vi "Funct img modulation core.vi"(8 "Pockels stay ON for at least this number of us after dwell time":dbl, 9 "Pockels turn ON at least this number of us before fill time completion":dbl, 11 "ROI setup":T1[](array[typedef]) {"Apparent Frame Size" format="%#_6f"; "Original FOV (um)" format="%#_6f"; "Pixels per miniscan" format="%#_6f"; "Dwell Time per pixel" format="%#_6f"; "Resolution" format="%#_6f"; "ROI group ID" format="%#_6f"; "Laser Power (%)" format="%#_6f"; "Zoom" format="%#_6f"; "Frame Size" format="%#_6f"; "Number of lines" format="%#_6f"; "Composite ID" format="%#_6f"; "Angle (deg)" format="%#_6f"; "ROI Time (ns)" format="%#_6f"; "ROI ID" format="%#_6f"; "Pixels in ROI" format="%#_6f"; "ROI index" format="%#_6f"; "Z stop" format="%#_6f"; "Y stop" format="%#_6f"; "X stop" format="%#_6f"; "Z start" format="%#_6f"; "X start" format="%#_6f"; "Y start" format="%#_6f"}) -> (1 "AO card sampling interval (us)":dbl=1.0 format="%#_13g us", 2 "Fill time (us)":dbl=24.4 format="%#_g us", 3 "waveform out":waveform(dbl), 5 "ROI Dwell Time (us)":dbl)   [LabVIEW 2020]
uses:
  User Interface/Visualisation/Functional Imaging Viewer/Typedefs/ROI parameters data type.ctl
  Typedefs/Rounding type.ctl
  Typedefs/Pockels modulation Internal cluster 1.ctl
  Global Variables/General Globals.vi
  Globals/gl_Pockels control globals.vi
  <vilib>/Waveform/WDTOps.llb/WDT Append Waveforms DBL.vi
panel:
  in  "Disable modulation":bool
  out "Pockels modulation signal":waveform(dbl)(graph)
  out "Remainder (us)":dbl
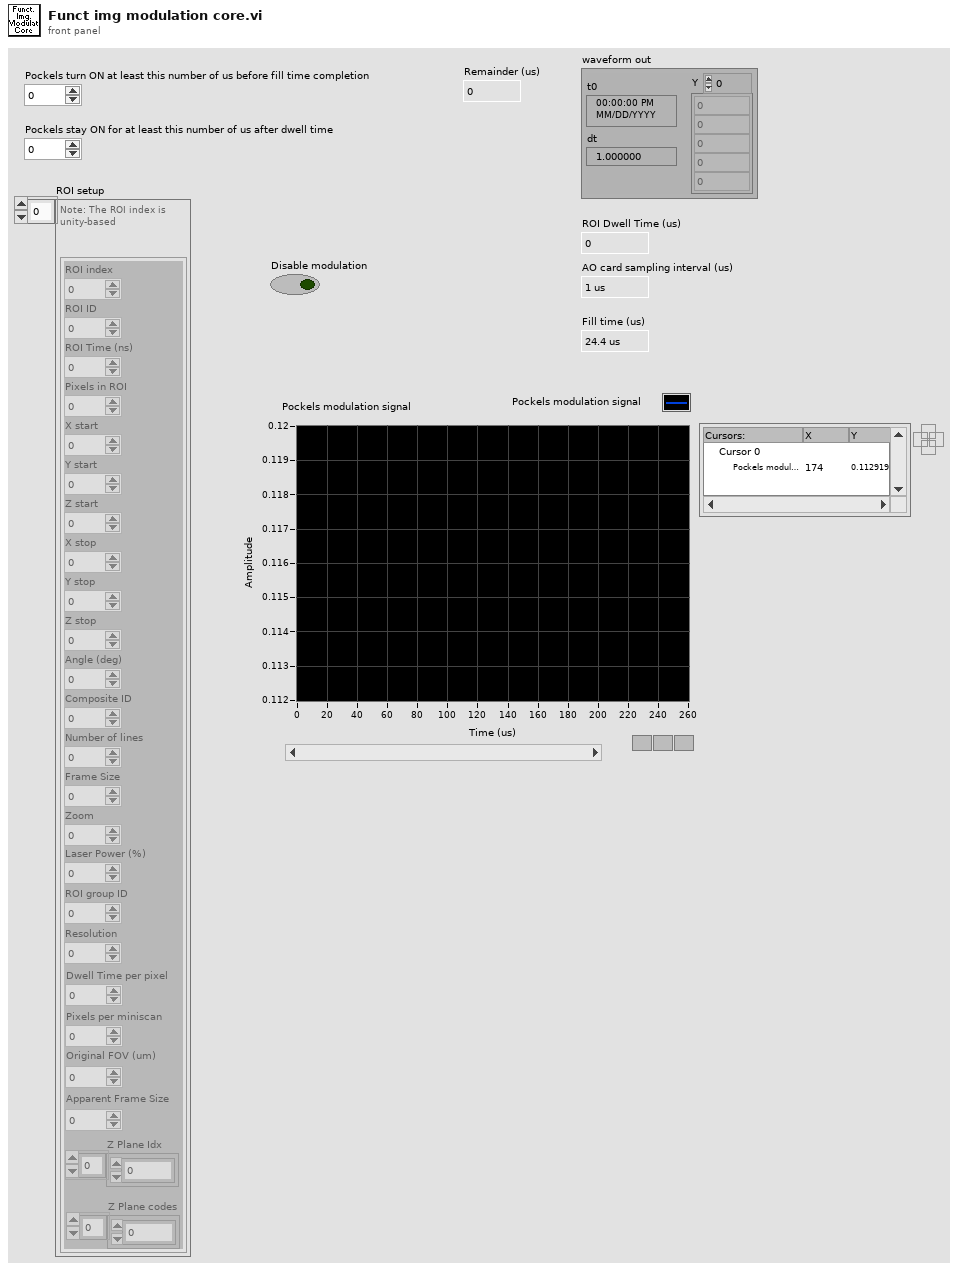
[diagram p1: front panel]
types:
  T1 = typedef "ROI parameters data type.ctl" = cluster{"ROI index":dbl, "ROI ID":dbl, "ROI Time (ns)":dbl, "Pixels in ROI":dbl, "X start":dbl, "Y start":dbl, "Z start":dbl, "X stop":dbl, "Y stop":dbl, "Z stop":dbl, "Angle (deg)":dbl, "Composite ID":dbl, "Number of lines":dbl, "Frame Size":dbl, "Zoom":dbl, "Laser Power (%)":dbl, "ROI group ID":dbl, "Resolution":dbl, "Dwell Time per pixel":dbl, "Pixels per miniscan":dbl, "Original FOV (um)":dbl, "Apparent Frame Size":dbl, "Z Plane Idx":i32[], "Z Plane codes":i32[]}
  T2 = enum16{"Movement correction is OFF", "Movement correction is ON"}
  T3 = typedef "Rounding type.ctl" = enum16{"No rounding", "Toward +Inf", "Toward -Inf"}
  T4 = typedef "Pockels modulation Internal cluster 1.ctl" = cluster{"Pockels ON \"Pre\" (samples)":i32, "Direction (+-Inf)":T3, "Additional duration to stay ON (samples)":i32, "Not the last ROI":bool}
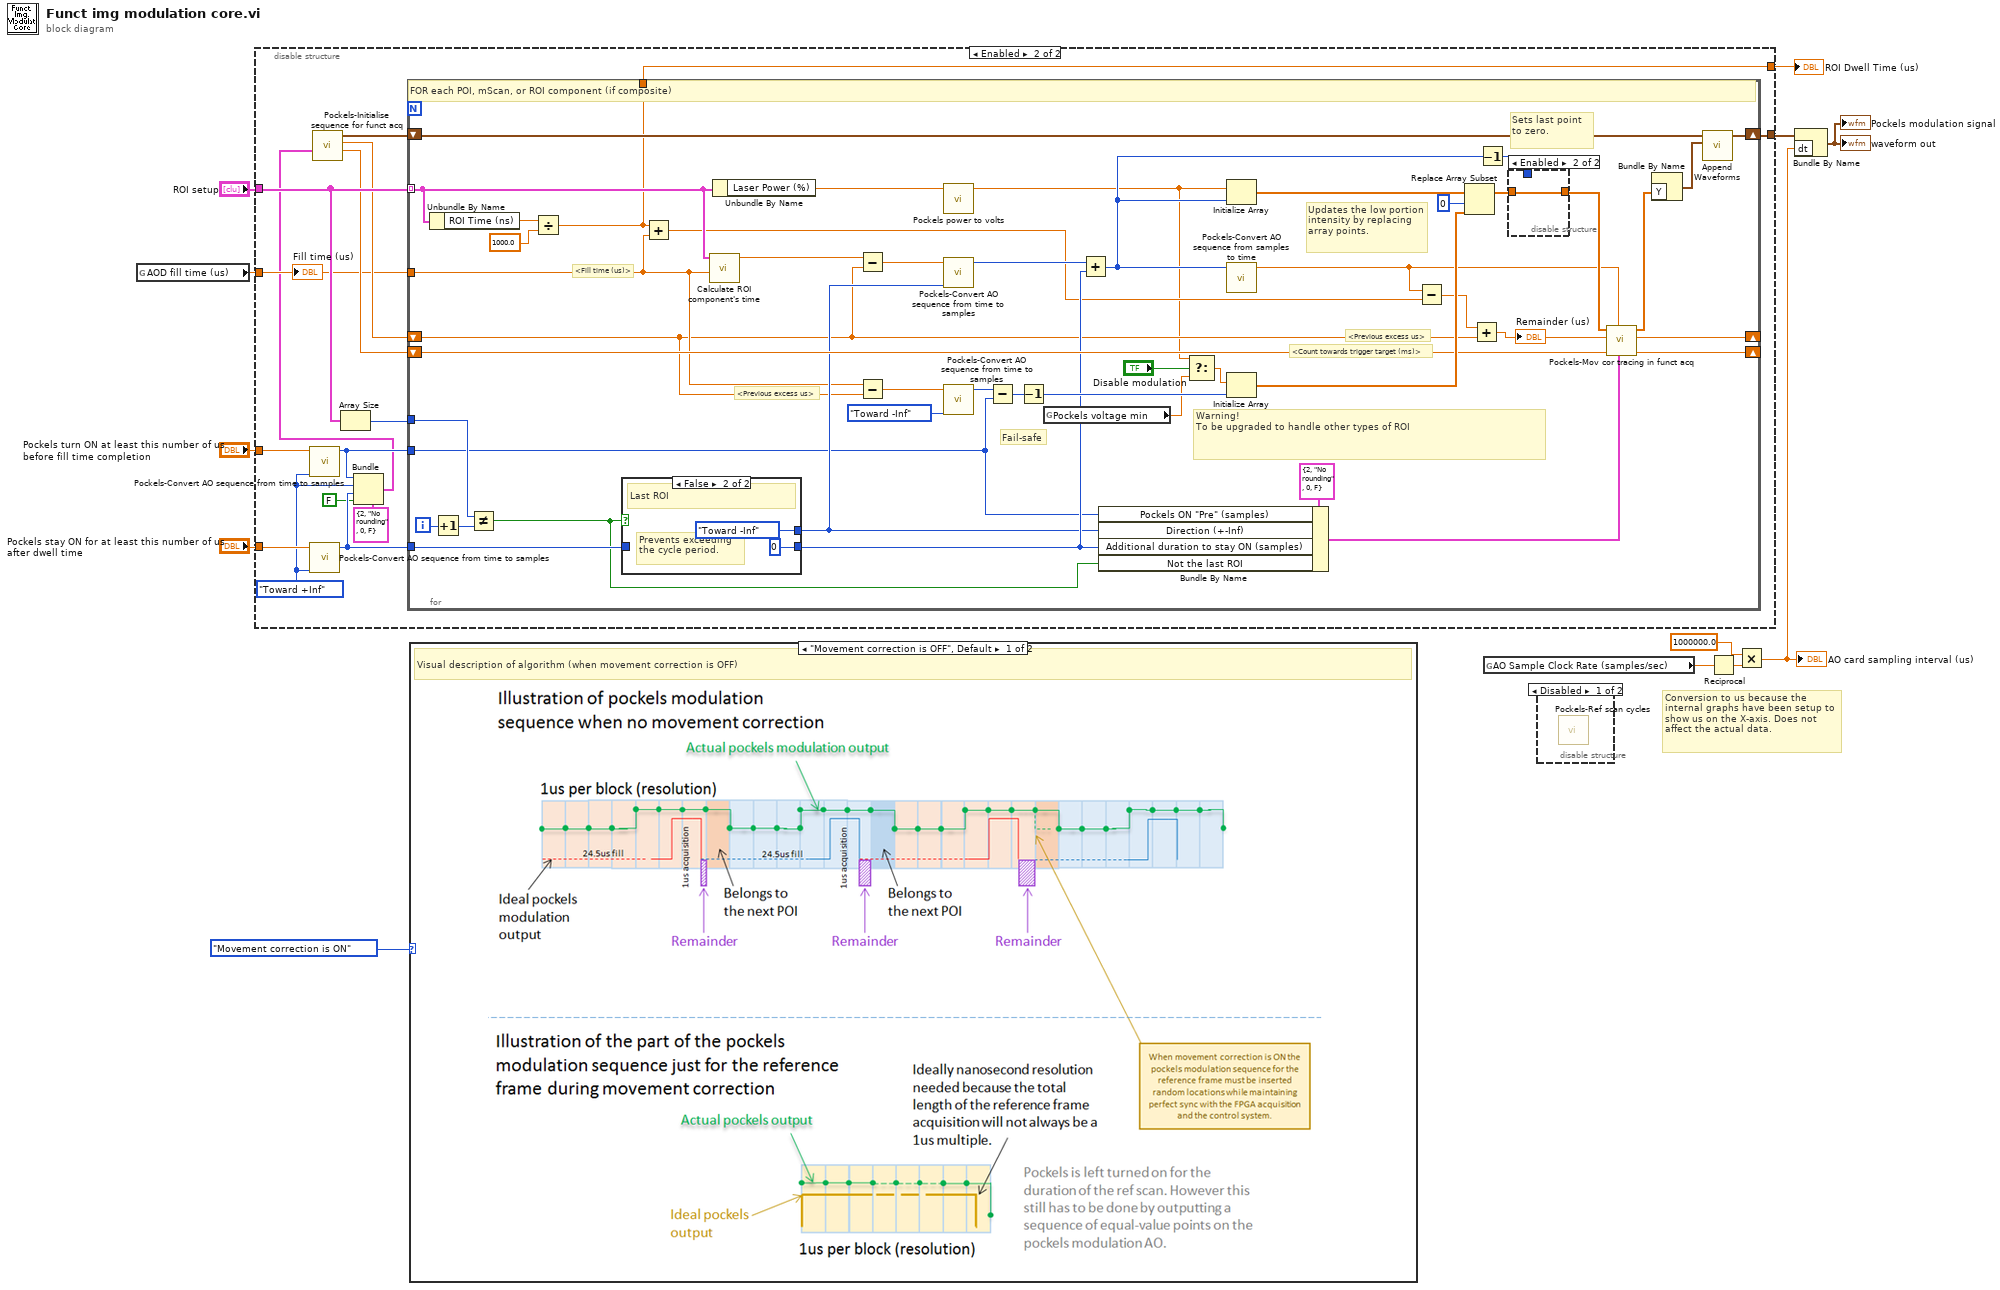
[diagram p0: block diagram]
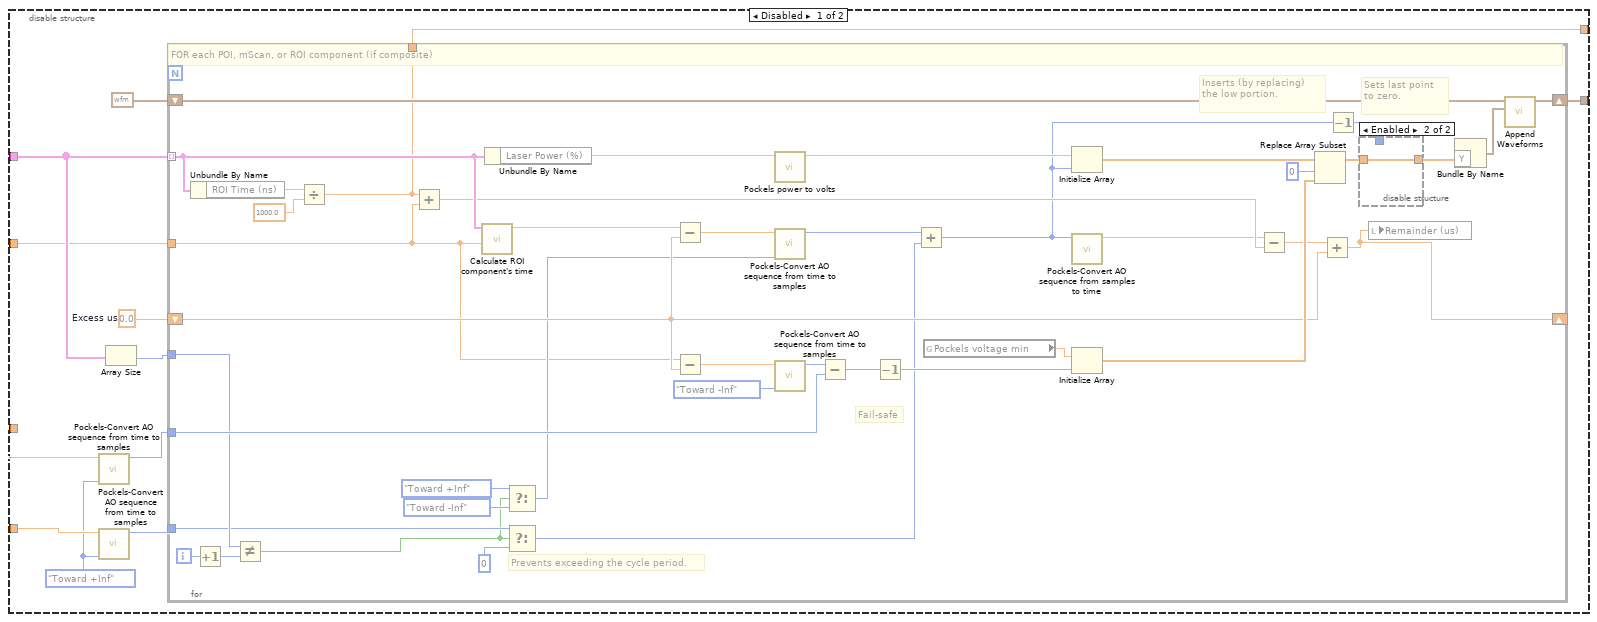
[diagram p3: hidden frame]
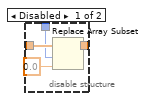
[diagram p4: hidden frame]
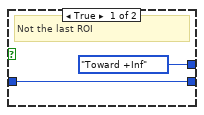
[diagram p5: hidden frame]
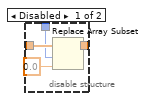
[diagram p6: hidden frame]
diagram:
  # "Conversion to us because the internal graphs have been setup to show us on the X-axis. Does not affect the actual data."
  n1 = global read "General Globals.vi" "AOD fill time (us)"() -> (w2:dbl)
  n2 = disable-structure shown="Enabled" {
    disable-tunnel: [w24 w87] -> w12
    disable-tunnel: "ROI setup" -> [w22 w85]
    disable-tunnel: w2 -> [w20 w78]
    disable-tunnel: [w19 w84] -> w8
    disable-tunnel: "Pockels stay ON for at least this number of us after dwell time" -> [w17 w83]
    disable-tunnel: "Pockels turn ON at least this number of us before fill time completion" -> [w15 w82]
    frame Disabled {
      w13 = Rounding_type."Toward +Inf" ("Direction (+Inf)")
      w21 = 0.0  # Excess us
      n3 = call "Pockels-Convert AO sequence from time to samples.vi"("Direction (+Inf)"=w13, "Duration of AO sequence (us)"=w15) -> ("Number of samples in AO sequence"=w14:i32)  [unwired: 9 in]
      n4 = call "Pockels-Convert AO sequence from time to samples.vi"("Direction (+Inf)"=w13, "Duration of AO sequence (us)"=w17) -> ("Number of samples in AO sequence"=w16:i32)  [unwired: 9 in]
      n5 = Array Size(array=w22) -> (size(s)=w23:i32)
      n6 = for {
        tunnel: w22 -> [w56] mode=indexing
        tunnel: w20 -> [w25]
        shift-right: [w51] -> w19
        shift-left: waveform(dbl) {"t0"=timestamp(0 s since 1904-01-01), "dt"=0.0, "Y"=[]} ("waveform out") -> [w62]
        tunnel: w16 -> [w32]
        tunnel: w14 -> [w57]
        shift-right: [w29] -> _
        shift-left: w21 -> [w35]
        tunnel: w23 -> [w41]
        tunnel: [w38] -> w24
        i -> [w43]
        # "Fail-safe"
        # "Prevents exceeding the cycle period."
        # "Inserts (by replacing) the low portion."
        # "Sets last point to zero."
        # "FOR each POI, mScan, or ROI component (if composite)"
        n7 = Unbundle By Name(w56) -> ("ROI Time (ns)"=w39:dbl)
        n8 = Increment(x=w43) -> (x+1=w42:i32)
        n9 = Not Equal?(x=w41, y=w42) -> (x != y?=w26:bool)
        n10 = Divide(x=w39, y=1000.0) -> (x/y=w38:dbl)
        n11 = Add(x=w38, y=w25) -> (x+y=w48:dbl)
        n12 = call "Calculate ROI component's time.vi"("AOD fill time (us)"=w25, "Normalised ROI setup"=w56) -> ("ROI component's time (us)"=w54:dbl)  [unwired: 9 in]
        n13 = Unbundle By Name(w56) -> ("Laser Power (%)"=w66:dbl)
        n14 = Select(t=Rounding_type."Toward +Inf" ("Direction (+Inf)"), s=w26, f=Rounding_type."Toward -Inf" ("Direction (+Inf)")) -> (s? t:f=w28:T3)
        n15 = Select(t=w32, s=w26, f=0) -> (s? t:f=w31:i32)
        n16 = Subtract(x=w54, y=w35) -> (x-y=w53:dbl)
        n17 = Subtract(x=w25, y=w35) -> (x-y=w52:dbl)
        n18 = call "Pockels power to volts.vi"("Pockels power (%)"=w66) -> ("Pockels control voltage (V)"=w65:dbl)  [unwired: 8 in, 2 out]
        n19 = call "Pockels-Convert AO sequence from time to samples.vi"("Direction (+Inf)"=w28, "Duration of AO sequence (us)"=w53) -> ("Number of samples in AO sequence"=w61:i32)  [unwired: 9 in]
        n20 = call "Pockels-Convert AO sequence from time to samples.vi"("Direction (+Inf)"=Rounding_type."Toward -Inf", "Duration of AO sequence (us)"=w52) -> ("Number of samples in AO sequence"=w60:i32)  [unwired: 9 in]
        n21 = Subtract(x=w60, y=w57) -> (x-y=w59:i32)
        n22 = Decrement(x=w59) -> (x-1=w58:i32)
        n23 = Add(x=w61, y=w31) -> (x+y=w34:i32)
        n24 = global read "gl_Pockels control globals.vi" "Pockels voltage min"() -> (w30:dbl)
        n25 = Initialize Array(w65, w34) -> (w45:dbl[])
        n26 = call "Pockels-Convert AO sequence from samples to time.vi"("Number of samples in AO sequence"=w34) -> ("Duration of AO sequence (us)"=w33:dbl)  [unwired: 10 in]
        n27 = Initialize Array(w30, w58) -> (w64:dbl[])
        n28 = Subtract(x=w33, y=w48) -> (x-y=w49:dbl)
        n29 = Replace Array Subset(array=w45, new element=w64, index=0) -> (w47:dbl[])
        n30 = Add(x=w49, y=w35) -> (x+y=w29:dbl)
        n31 = Decrement(x=w34) -> (x-1=w44:i32)
        n32 = disable-structure shown="Enabled" {
          disable-tunnel: w47 -> [w70 w71]
          disable-tunnel: [w69 w71] -> w46
          disable-tunnel: w44 -> [w67 _]
          frame Disabled {
            n33 = Replace Array Subset(array=w70, new element=0.0 ("new element/subarray"), index=w67) -> (w69:dbl[])
          }
          frame Enabled {
          }
        }
        n34 = local write "Remainder (us)"(w29) -> ()
        n35 = Bundle By Name("Y"=w46) -> (w50:waveform(dbl))  [unwired: 1 in]
        n36 = call-poly <vilib>:"Append Waveforms.vi"("waveform B"=w50, "waveform A"=w62) -> ("waveform out"=w51:waveform(dbl))  [unwired: 8 in, 1 out]
      }
    }
    frame Enabled {
      w76 = Rounding_type."Toward +Inf" ("Direction (+Inf)")
      n37 = call "Pockels-Convert AO sequence from time to samples.vi"("Direction (+Inf)"=w76, "Duration of AO sequence (us)"=w82) -> ("Number of samples in AO sequence"=w77:i32)  [unwired: 9 in]
      n38 = call "Pockels-Convert AO sequence from time to samples.vi"("Direction (+Inf)"=w76, "Duration of AO sequence (us)"=w83) -> ("Number of samples in AO sequence"=w75:i32)  [unwired: 9 in]
      n39 = Array Size(array=w85) -> (size(s)=w86:i32)
      n40 = Bundle(cluster=T4 {"Pockels ON \"Pre\" (samples)"=2, "Direction (+-Inf)"=enum."No rounding", "Additional duration to stay ON (samples)"=0, "Not the last ROI"=FALSE} ("output cluster"), "Pockels ON \"Pre\" (samples)"=w77, "Direction (+-Inf)"=w76, "Additional duration to stay ON (samples)"=w75, "Not the last ROI"=FALSE ("Last ROI reached")) -> (w74:T4)
      n41 = call "Pockels-Initialise sequence for funct acq.vi"("Cluster"=w74) -> ("Count towards trigger target (ms)"=w80:dbl, "Excess (us)"=w79:dbl, "waveform out"=w81:waveform(dbl))  [unwired: 8 in]
      n42 = for {
        tunnel: w85 -> [w126] mode=indexing
        shift-right: [w121] -> w84
        shift-left: w81 -> [w131]
        tunnel: w75 -> [w109]
        tunnel: w77 -> [w95]
        shift-right: [w106] -> _
        shift-left: w79 -> [w96]
        tunnel: w86 -> [w113]
        tunnel: [w111] -> w87
        shift-right: [w103] -> _
        shift-left: w80 -> [w104]
        tunnel: w78 -> [w97]
        i -> [w115]
        # "Updates the low portion intensity by replacing array points."
        # "<Previous excess us>"
        # "<Fill time (us)>"
        # "Warning!\nTo be upgraded to handle other types of ROI"
        # "<Previous excess us>"
        # "<Count towards trigger target (ms)>"
        # "Fail-safe"
        # "Sets last point to zero."
        # "FOR each POI, mScan, or ROI component (if composite)"
        n43 = Unbundle By Name(w126) -> ("ROI Time (ns)"=w112:dbl)
        n44 = Increment(x=w115) -> (x+1=w114:i32)
        n45 = Not Equal?(x=w113, y=w114) -> (x != y?=w92:bool)
        n46 = Divide(x=w112, y=1000.0) -> (x/y=w111:dbl)
        n47 = case shown="False" w92 {
          tunnel: [Rounding_type."Toward +Inf" ("Direction (+Inf)") Rounding_type."Toward -Inf" ("Direction (+Inf)")] -> w99
          tunnel: w109 -> [w136 _]
          tunnel: [w136 0 ("f")] -> w102
          frame True {
            # "Not the last ROI"
          }
          frame False {
            # "Prevents exceeding the cycle period."
            # "Last ROI"
          }
        }
        n48 = Add(x=w111, y=w97) -> (x+y=w94:dbl)
        n49 = call "Calculate ROI component's time.vi"("AOD fill time (us)"=w97, "Normalised ROI setup"=w126) -> ("ROI component's time (us)"=w124:dbl)  [unwired: 9 in]
        n50 = Unbundle By Name(w126) -> ("Laser Power (%)"=w134:dbl)
        n51 = Subtract(x=w124, y=w96) -> (x-y=w123:dbl)
        n52 = Subtract(x=w97, y=w96) -> (x-y=w122:dbl)
        n53 = call "Pockels power to volts.vi"("Pockels power (%)"=w134) -> ("Pockels control voltage (V)"=w89:dbl)  [unwired: 8 in, 2 out]
        n54 = call "Pockels-Convert AO sequence from time to samples.vi"("Direction (+Inf)"=w99, "Duration of AO sequence (us)"=w123) -> ("Number of samples in AO sequence"=w130:i32)  [unwired: 9 in]
        n55 = call "Pockels-Convert AO sequence from time to samples.vi"("Direction (+Inf)"=Rounding_type."Toward -Inf", "Duration of AO sequence (us)"=w122) -> ("Number of samples in AO sequence"=w129:i32)  [unwired: 9 in]
        n56 = Subtract(x=w129, y=w95) -> (x-y=w128:i32)
        n57 = Decrement(x=w128) -> (x-1=w127:i32)
        n58 = global read "gl_Pockels control globals.vi" "Pockels voltage min"() -> (w91:dbl)
        n59 = Add(x=w130, y=w102) -> (x+y=w110:i32)
        n60 = Bundle By Name(cluster=T4 {"Pockels ON \"Pre\" (samples)"=2, "Direction (+-Inf)"=enum."No rounding", "Additional duration to stay ON (samples)"=0, "Not the last ROI"=FALSE} ("output cluster"), "Pockels ON \"Pre\" (samples)"=w95, "Direction (+-Inf)"=w99, "Additional duration to stay ON (samples)"=w102, "Not the last ROI"=w92) -> (w100:T4)
        n61 = Select(t=w89, s="Disable modulation", f=w91) -> (s? t:f=w90:dbl)
        n62 = Initialize Array(w89, w110) -> (w117:dbl[])
        n63 = call "Pockels-Convert AO sequence from samples to time.vi"("Number of samples in AO sequence"=w110) -> ("Duration of AO sequence (us)"=w93:dbl)  [unwired: 10 in]
        n64 = Initialize Array(w90, w127) -> (w133:dbl[])
        n65 = Subtract(x=w93, y=w94) -> (x-y=w119:dbl)
        n66 = Replace Array Subset(array=w117, new element=w133, index=0) -> (w118:dbl[])
        n67 = Add(x=w119, y=w96) -> (x+y=w105:dbl)
        "Remainder (us)" <- w105
        n68 = Decrement(x=w110) -> (x-1=w116:i32)
        n69 = disable-structure shown="Enabled" {
          disable-tunnel: w118 -> [w142 w143]
          disable-tunnel: [w141 w143] -> w107
          disable-tunnel: w116 -> [w139 _]
          frame Disabled {
            n70 = Replace Array Subset(array=w142, new element=0.0 ("new element/subarray"), index=w139) -> (w141:dbl[])
          }
          frame Enabled {
          }
        }
        n71 = call "Pockels-Mov cor tracing in funct acq.vi"("Cluster"=w100, "Actual component time (us)"=w93, "Count towards trigger target (ms) in"=w104, "Excess (us) in"=w105, "Single ROI pockels modulation AO sequence (in)"=w107) -> ("Count towards trigger target (ms)"=w103:dbl, "Excess (us)"=w106:dbl, "AO pockels modulation sequence (out)"=w108:dbl[])  [unwired: 4 in]
        n72 = Bundle By Name("Y"=w108) -> (w120:waveform(dbl))  [unwired: 1 in]
        n73 = call-poly <vilib>:"Append Waveforms.vi"("waveform B"=w120, "waveform A"=w131) -> ("waveform out"=w121:waveform(dbl))  [unwired: 8 in, 1 out]
      }
      "Fill time (us)" <- w78
    }
  }
  "ROI Dwell Time (us)" <- w12
  n74 = case shown="\"Movement correction is OFF\", Default" T2."Movement correction is ON" ("Enum") {
    frame "Movement correction is OFF", Default {
      # "Visual description of algorithm (when movement correction is OFF)"
    }
    frame "Movement correction is ON" {
      # "Visual description of algorithm (when movement correction is ON)"
    }
  }
  n75 = global read "General Globals.vi" "AO Sample Clock Rate (samples/sec)"() -> (w9:dbl)
  n76 = disable-structure shown="Disabled" {
    frame Disabled {
      n77 = call "Pockels-Ref scan cycles.vi"() -> ()  [unwired: 10 in, 2 out]
    }
    frame Enabled {
    }
  }
  n78 = Reciprocal(x=w9) -> (1/x=w10:dbl)
  n79 = Multiply(x=1000000.0, y=w10) -> (x*y=w7:dbl)
  "AO card sampling interval (us)" <- w7
  n80 = Bundle By Name(cluster=w8, "dt"=w7) -> (→"waveform out" →"Pockels modulation signal":waveform(dbl))
